vi "Push All Control Parameters.vi"(6 "error in":errorcluster, 7 "Manlight VISA Refnum":refnum<visa-resource-name>, 8 "Enabled Hardware":T1={"Confocal"=TRUE, "Pinhole"=FALSE, "PIFOC"=TRUE, "Manlight"=FALSE, "iFlex"=FALSE}, 9 "All Controlls For Savinge":T2={"Confocal Controls"={"Channel Selection"=enum."A", "Pixel Count"={"Pixels in X"=512, "Pixels in Y"=512}, "Field Size"=50.0, "Frames"=2, "Averaging"=FALSE, "Alignment"=0.0, "Scan Mode"=TRUE, "Gain"={"Gain A"=1, "Gain B"=1}, "Enable PMTs"={"A"=TRUE, "B"=TRUE}, "Voltage Range"={"Range A"=10, "Range B"=10}, "Multi Frame Count"=0.0, "Trigger Mode"=2.0, "Real Time Averaging"=TRUE, "PFOV"=0.0, "MicronsPerPx"=0.0}, "iFlex Control"={"Power 561"=0.0, "Power 488"=0.0, "Global Shutter"=FALSE, "561 Shutter"=FALSE}, "PIFOC Settings"={"PIFOC Position (mm) [SET]"=0.0, "PIFOC Position\n(um) [ACT]"=0.0087, "last command"=""}, "PinSelector"=6.0, "Manlight Controls"={"Manlight Power"=0.0, "Open Serial"=FALSE, "VISA Refnum"=""}, "Exp Params"={"Experiment Type"="2D Snapshot", "Experiment Name"="Experiment_1", "ExpPath"=path "E:/Data", "TSFrames"=1000, "TSfps"=1000, "ZTSFrames"=1000, "ZTSdt"=1, "Streaming"=FALSE, "Z Stack Settings"={"Start"=0.0, "Step Size"=0.1, "Finish"=1.0}, "total images"=1, "tdms ref"=refnum, "frame #"=0, "images per stack"=1, "total stacks"=1, "period"=1, "PI MVR Increment"=""}} {"Exp Params"."period" min=1; "Exp Params"."total stacks" min=1; "Exp Params"."images per stack" min=1; "Exp Params"."total images" min=1; "Exp Params"."Z Stack Settings"."Start" min=0.0 max=100.0 step=0.1; "Exp Params"."Z Stack Settings"."Step Size" min=0.1 max=100.0 step=0.1; "Exp Params"."Z Stack Settings"."Finish" min=0.0 max=100.0 step=0.1; "Exp Params"."TSFrames" min=1 step=1; "Exp Params"."ZTSdt" min=1 step=1; "Exp Params"."ZTSFrames" min=2 step=1; "Exp Params"."TSfps" min=1 max=1000 step=1; "Manlight Controls"."Manlight Power" min=0.0 max=10.0 step=0.1 scale=0.0..10.0; "PinSelector" items=["25", "30", "35", "40", "45", "50", "60", "70", "80", "90", "100", "125", "200", "300", "1000", "2000"]; "PIFOC Settings"."PIFOC Position\n(um) [ACT]" format="%.2f"; "PIFOC Settings"."PIFOC Position (mm) [SET]" min=0.0 max=100.0 step=0.1 scale=0.0..100.0; "iFlex Control"."Power 561" min=12.5 max=100.0 step=0.1 scale=0.0..100.0; "iFlex Control"."Power 488" min=30.0 max=100.0 step=0.1 scale=0.0..100.0; "Confocal Controls"."Field Size" min=5.0 max=255.0 step=1.0 scale=5.0..255.0; "Confocal Controls"."PFOV" min=1.0 max=300.0 step=0.1; "Confocal Controls"."MicronsPerPx" min=0.01 step=0.01 format="%.2f"; "Confocal Controls"."Gain"."Gain B" min=1 max=100 step=1; "Confocal Controls"."Gain"."Gain A" min=1 max=100 step=1; "Confocal Controls"."Voltage Range"."Range B" items=["100mV"=5, "200mV"=6, "400mV"=7, "1V"=10, "2V"=11, "4V"=12]; "Confocal Controls"."Voltage Range"."Range A" items=["100mV"=5, "200mV"=6, "400mV"=7, "1V"=10, "2V"=11, "4V"=12]; "Confocal Controls"."Pixel Count"."Pixels in Y" items=["32"=32, "64"=64, "128"=128, "256"=256, "512"=512, "1024"=1024, "2048"=2048]; "Confocal Controls"."Pixel Count"."Pixels in X" items=["32"=32, "64"=64, "128"=128, "256"=256, "512"=512, "1024"=1024, "2048"=2048]}) -> (0 "error out":errorcluster)   [LabVIEW 2020]
uses:
  _Controls/All Controls For Saving.ctl
  _Controls/Confocal Controls.ctl
  _Controls/iFlex.ctl
  _Controls/PIFOC Position.ctl
  _Controls/Manlight Controls.ctl
  _Controls/Exp Params.ctl
  _Globals/Global Controls.vi
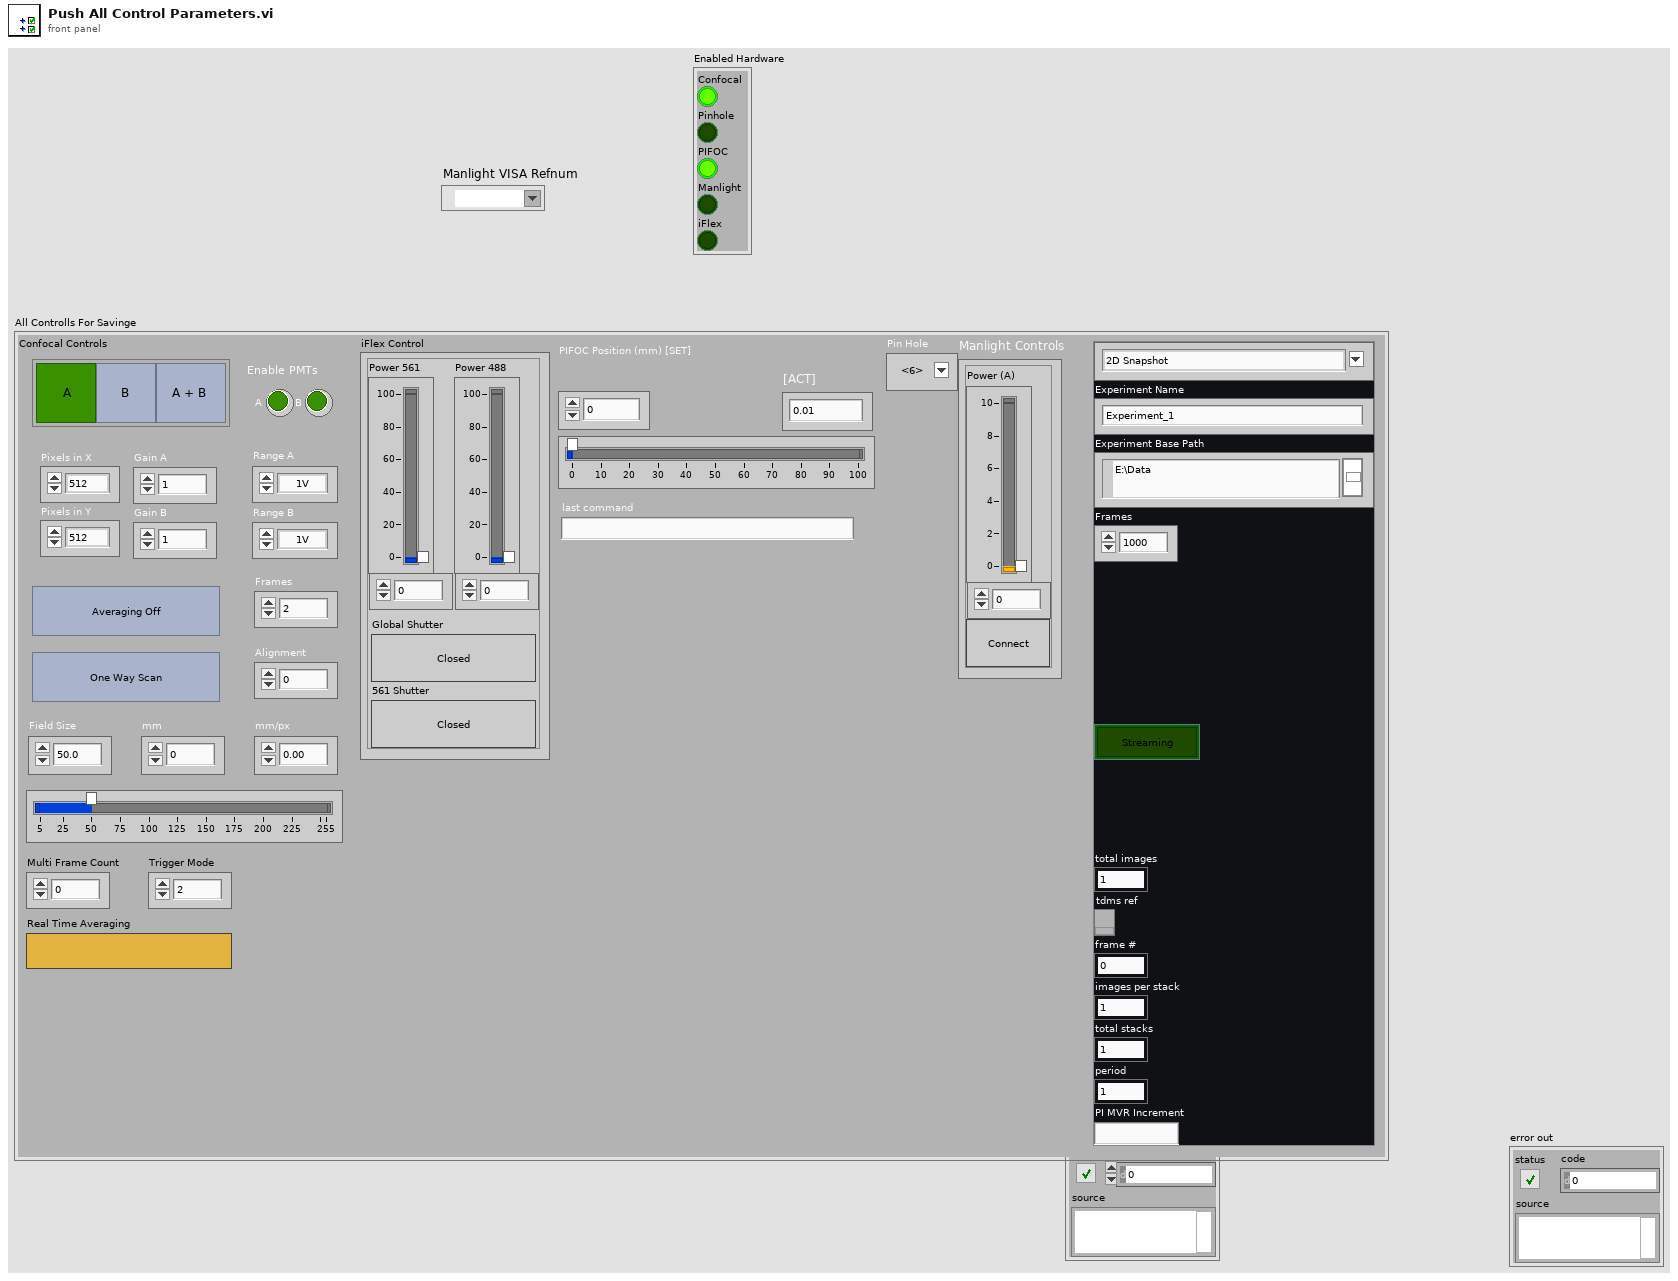
[diagram p1: front panel]
types:
  T1 = cluster{"Confocal":bool, "Pinhole":bool, "PIFOC":bool, "Manlight":bool, "iFlex":bool}
  T2 = typedef "All Controls For Saving.ctl" = cluster{"Confocal Controls":T3, "iFlex Control":T4, "PIFOC Settings":T5, "PinSelector":dbl, "Manlight Controls":T6, "Exp Params":T7}
  T3 = typedef "Confocal Controls.ctl" = cluster{"Channel Selection":enum32{"A", "B", "AB"}, "Pixel Count":cluster{"Pixels in X":u32, "Pixels in Y":u32}, "Field Size":dbl, "Frames":u8, "Averaging":bool, "Alignment":dbl, "Scan Mode":bool, "Gain":cluster{"Gain A":u8, "Gain B":u8}, "Enable PMTs":cluster{"A":bool, "B":bool}, "Voltage Range":cluster{"Range A":u16, "Range B":u16}, "Multi Frame Count":dbl, "Trigger Mode":dbl, "Real Time Averaging":bool, "PFOV":dbl, "MicronsPerPx":dbl}
  T4 = typedef "iFlex.ctl" = cluster{"Power 561":dbl, "Power 488":dbl, "Global Shutter":bool, "561 Shutter":bool}
  T5 = typedef "PIFOC Position.ctl" = cluster{"PIFOC Position (mm) [SET]":dbl, "PIFOC Position\n(um) [ACT]":dbl, "last command":string}
  T6 = typedef "Manlight Controls.ctl" = cluster{"Manlight Power":dbl, "Open Serial":bool, "VISA Refnum":refnum<visa-resource-name>}
  T7 = typedef "Exp Params.ctl" = cluster{"Experiment Type":string, "Experiment Name":string, "ExpPath":path, "TSFrames":i32, "TSfps":i32, "ZTSFrames":i32, "ZTSdt":i32, "Streaming":bool, "Z Stack Settings":cluster{"Start":dbl, "Step Size":dbl, "Finish":dbl}, "total images":i32, "tdms ref":refnum<k34>, "frame #":i64, "images per stack":i32, "total stacks":i32, "period":i32, "PI MVR Increment":string}
  T8 = typedef "Tweezertron Ctrl Refs.ctl" = cluster{"LSM Settings":refnum<vi>, "iFlex Control":refnum<vi>, "PIFOC Settings":refnum<vi>, "PinSelector":refnum<vi>, "Manlight Controls":refnum<vi>, "Exp Params":refnum<vi>, "Image Thresholds":refnum<vi>}
  T9 = enum8{"Enabled", "Disabled", "Disabled and Grayed Out"}
  T10 = cluster{"iFlex Control":T4, "index of change":i32[]}
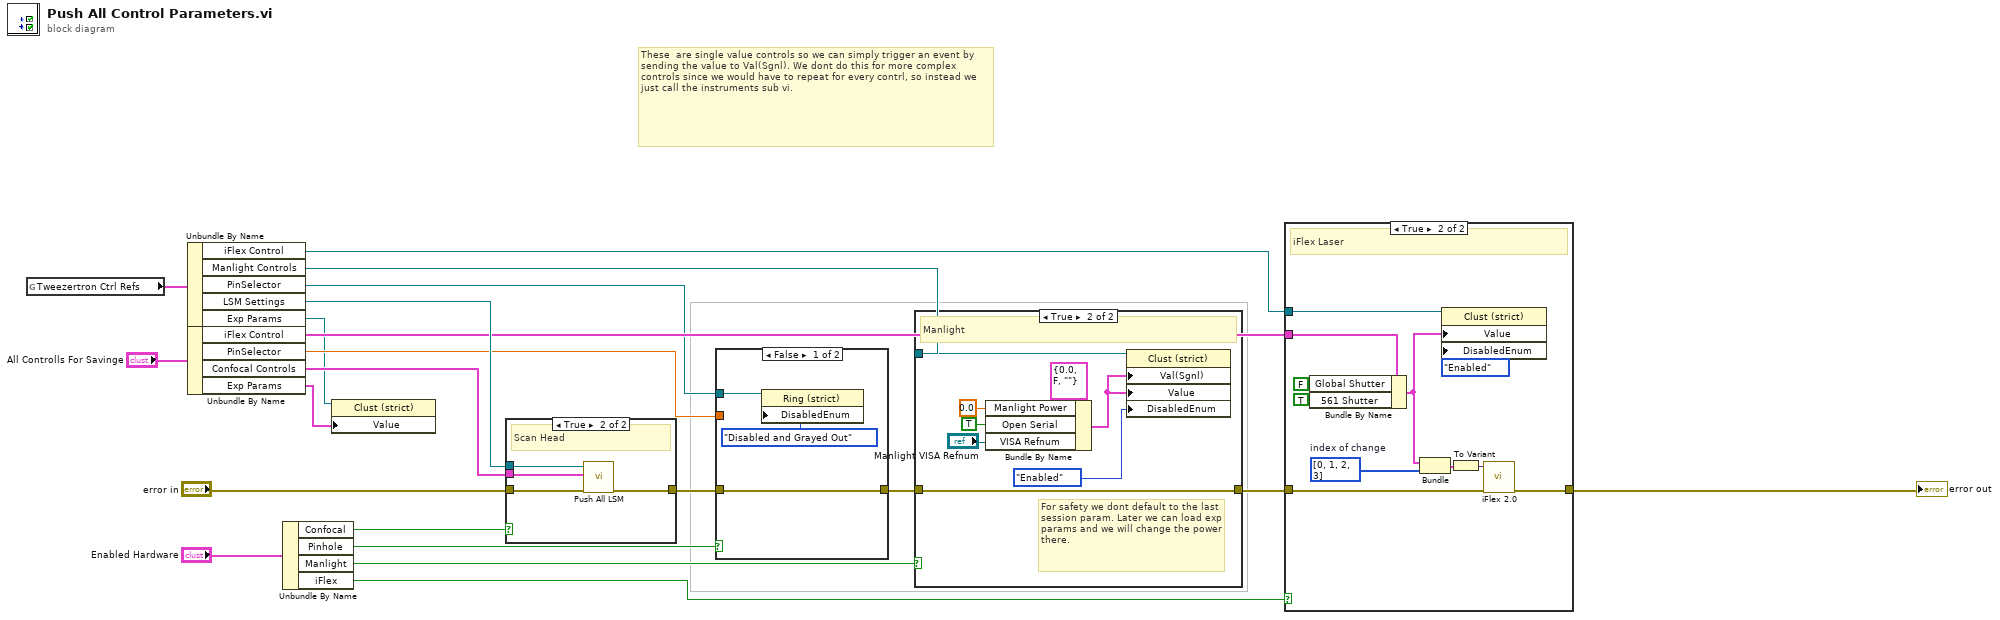
[diagram p0: block diagram]
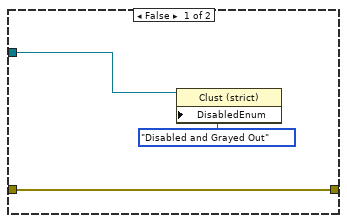
[diagram p2: hidden frame]
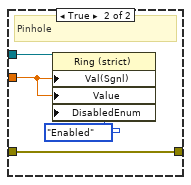
[diagram p3: hidden frame]
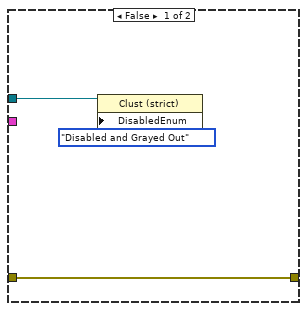
[diagram p4: hidden frame]
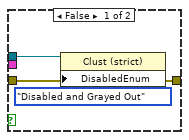
[diagram p5: hidden frame]
diagram:
  # "These  are single value controls so we can simply trigger an event by sending the value to Val(Sgnl). We dont do this for more complex controls since we would have to repeat for every contrl, so instead we just call the instruments sub vi."
  n1 = global read "Global Controls.vi" "Tweezertron Ctrl Refs"() -> (w9:T8)
  n2 = Unbundle By Name(w9) -> ("iFlex Control"=w10:refnum<vi>, "Manlight Controls"=w4:refnum<vi>, "PinSelector"=w5:refnum<vi>, "LSM Settings"=w18:refnum<vi>, "Exp Params"=w2:refnum<vi>)
  n3 = Unbundle By Name("All Controlls For Savinge") -> ("iFlex Control"=w12:T4, "PinSelector"=w11:dbl, "Confocal Controls"=w19:T3, "Exp Params"=w1:T7)
  n4 = Unbundle By Name("Enabled Hardware") -> ("Confocal"=w16:bool, "Pinhole"=w14:bool, "Manlight"=w7:bool, "iFlex"=w8:bool)
  n5 = property class="Clust (strict)"(reference=w2, "Value"=w1) -> ()  [unwired: 1 in, 2 out]
  n6 = case shown="True" w16 {
    tunnel: "error in" -> [w24 w28]
    tunnel: w19 -> [_ w27]
    tunnel: w18 -> [w22 w26]
    tunnel: [w24 w25] -> w13
    frame False {
      n7 = property class="Clust (strict)"(reference=w22, "DisabledEnum"=T9."Disabled and Grayed Out" ("Disabled")) -> ()  [unwired: 1 in, 2 out]
    }
    frame True {
      # "Scan Head"
      n8 = call "Push All LSM.vi"("error in (no error)"=w28, "Confocal Controls"=w27, "LSM Ctrls Ref"=w26) -> ("error out"=w25:errorcluster)  [unwired: 8 in]
    }
  }
  n9 = case shown="False" w14 {
    tunnel: w13 -> [w31 w33]
    tunnel: w11 -> [_ w34]
    tunnel: w5 -> [w30 w35]
    tunnel: [w31 w33] -> w6
    frame False {
      n10 = property class="Ring (strict)"(reference=w30, "DisabledEnum"=T9."Disabled and Grayed Out" ("Disabled")) -> ()  [unwired: 1 in, 2 out]
    }
    frame True {
      # "Pinhole"
      n11 = property class="Ring (strict)"(reference=w35, "Val(Sgnl)"=w34, "Value"=w34, "DisabledEnum"=T9."Enabled" ("Disabled")) -> ()  [unwired: 1 in, 2 out]
    }
  }
  n12 = case shown="True" w7 {
    tunnel: w6 -> [w38 w45]
    tunnel: w4 -> [w37 w46]
    tunnel: [w38 w45] -> w3
    frame False {
      n13 = property class="Clust (strict)"(reference=w37, "DisabledEnum"=T9."Disabled and Grayed Out" ("Disabled")) -> ()  [unwired: 1 in, 2 out]
    }
    frame True {
      # "For safety we dont default to the last session param. Later we can load exp params and we will change the power there."
      # "Manlight"
      n14 = Bundle By Name(cluster=T6 {"Manlight Power"=0.0, "Open Serial"=FALSE, "VISA Refnum"=""} ("Manlight Controls"), "Manlight Power"=0.0, "Open Serial"=TRUE, "VISA Refnum"="Manlight VISA Refnum") -> (w39:T6)
      n15 = property class="Clust (strict)"(reference=w46, "Val(Sgnl)"=w39, "Value"=w39, "DisabledEnum"=T9."Enabled" ("Disabled")) -> ()  [unwired: 1 in, 2 out]
    }
  }
  n16 = case shown="True" w8 {
    tunnel: w3 -> [w49 w57]
    tunnel: w10 -> [w48 w56]
    tunnel: [w49 w55] -> w17
    tunnel: w12 -> [_ w54]
    frame False {
      n17 = property class="Clust (strict)"(reference=w48, "DisabledEnum"=T9."Disabled and Grayed Out" ("Disabled")) -> ()  [unwired: 1 in, 2 out]
    }
    frame True {
      w58 = i32[] [0, 1, 2, 3]  # index of change
      # "iFlex Laser"
      n18 = Bundle By Name(cluster=w54, "Global Shutter"=FALSE, "561 Shutter"=TRUE) -> (w51:T4)
      n19 = Bundle("iFlex Control"=w51, "index of change"=w58) -> (w59:T10)  [unwired: 1 in]
      n20 = property class="Clust (strict)"(reference=w56, "Value"=w51, "DisabledEnum"=T9."Enabled" ("Disabled")) -> ()  [unwired: 1 in, 2 out]
      n21 = To Variant(anything=w59) -> (Variant=w60:variant)
      n22 = call "iFlex 2.0 .vi"("error in"=w57, "params"=w60) -> ("error out"=w55:errorcluster)  [unwired: 9 in]
    }
  }
  "error out" <- w17
